vi "gjson_UniqueNames.vi"(8 "error in":errorcluster, 11 "Cluster Elements":variant[](array[variant])) -> (0 "error out":errorcluster, 3 "Cluster Elements Out":variant[](array[variant]))   [LabVIEW 2015, in "Json2Labv.lvlib"]
doc: "Ensures no two elements of the same hierarchy have the same name."
uses:
  Json2Labv.lvlib
  <vilib>/Utility/VariantDataType/VariantType.lvlib
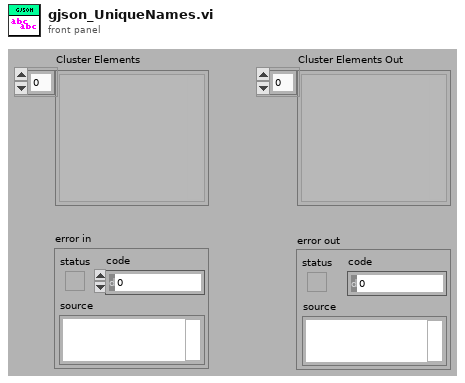
[diagram p1: front panel]
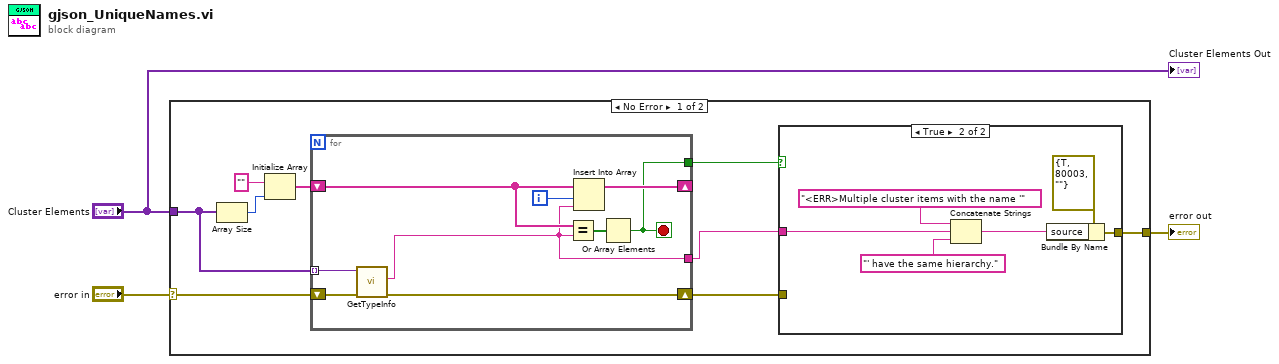
[diagram p0: block diagram]
diagram:
  n1 = case shown="No Error" "error in" {
    selector: "error in" -> [w5 w29]
    tunnel: "Cluster Elements" -> [w11 _]
    tunnel: [w6 w29] -> w2
    frame No Error {
      n2 = Array Size(array=w11) -> (size(s)=w10:i32)
      n3 = Initialize Array("", w10) -> (w9:string[])
      n4 = for {
        tunnel: w11 -> [w28] mode=indexing
        shift-right: [w21] -> w7
        shift-left: w5 -> [w27]
        shift-right: [w26] -> _
        shift-left: w9 -> [w24]
        tunnel: [w20] -> w4
        tunnel: [w22] -> w8
        i -> [w25]
        stop <- w22 stop-if-true
        n5 = call <vilib>:"GetTypeInfo.vi"("error in (no error)"=w27, "Variant"=w28) -> ("error out"=w21:errorcluster, "Name"=w20:string)  [unwired: 5 in, 3 out]
        n6 = Equal?(x=w24, y=w20) -> (x = y?=w23:bool[])
        n7 = Insert Into Array(array=w24, index=w25, new element=w20) -> (w26:string[])
        n8 = Or Array Elements(Boolean array=w23) -> (logical OR=w22:bool)
      }
      n9 = case shown="True" w8 {
        tunnel: w7 -> [w13 _]
        tunnel: [w13 w18] -> w6
        tunnel: w4 -> [_ w14]
        frame False {
        }
        frame True {
          n10 = Concatenate Strings("<ERR>Multiple cluster items with the name '", w14, "' have the same hierarchy.") -> (w15:string)
          n11 = Bundle By Name(cluster=errorcluster {"status"=TRUE, "code"=80003, "source"=""} ("error in"), "source"=w15) -> (w18:errorcluster)
        }
      }
    }
    frame Error {
    }
  }
  "error out" <- w2
  "Cluster Elements Out" <- "Cluster Elements"
